vi "STOP ALL.vi"(0 "reference in":refnum<class "PM_Group.lvclass">, 5 "error in (no error)":errorcluster) -> (14 "reference out":refnum<class "PM_Group.lvclass">, 19 "error out":errorcluster)   [LabVIEW 2019, in "PM_Group.lvclass"]
uses:
  PM_Group.lvclass
  PM_Group.lvclass/PM_Group.ctl
  Engine_1DO_2DI_class/Engine_1DO_2DI.lvclass
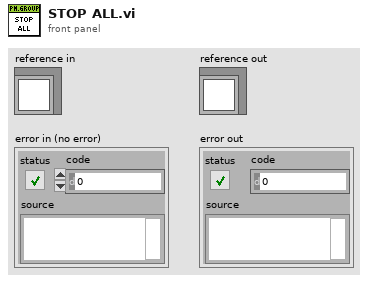
[diagram p1: front panel]
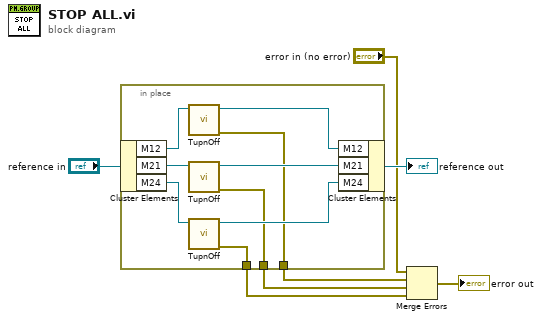
[diagram p0: block diagram]
diagram:
  n1 = in-place {
    in-place-border: [w10] -> w2
    in-place-border: [w9] -> w3
    in-place-border: [w8] -> w4
    n2 = in-place-cluster #1("reference in") -> ("M12"=w16:refnum<class "Engine_1DO_2DI.lvclass">, "M21"=w15:refnum<class "Engine_1DO_2DI.lvclass">, "M24"=w14:refnum<class "Engine_1DO_2DI.lvclass">)
    n3 = call "TupnOff.vi"("Pump_1AI_1DO_2DI in"=w16) -> ("error out"=w8:errorcluster, "Pump_1AI_1DO_2DI out"=w13:refnum<class "Engine_1DO_2DI.lvclass">)  [unwired: 9 in]
    n4 = call "TupnOff.vi"("Pump_1AI_1DO_2DI in"=w15) -> ("error out"=w9:errorcluster, "Pump_1AI_1DO_2DI out"=w12:refnum<class "Engine_1DO_2DI.lvclass">)  [unwired: 9 in]
    n5 = call "TupnOff.vi"("Pump_1AI_1DO_2DI in"=w14) -> ("error out"=w10:errorcluster, "Pump_1AI_1DO_2DI out"=w11:refnum<class "Engine_1DO_2DI.lvclass">)  [unwired: 9 in]
    n6 = in-place-cluster #1("M12"=w13, "M21"=w12, "M24"=w11) -> (→"reference out":refnum<class "PM_Group.lvclass">)
  }
  n7 = Merge Errors("error in (no error)", w4, w3, w2) -> (→"error out":errorcluster)
